vi "BRig_dataExp_T_Reward_min_L.vi"() -> (2 "output_Tcycle_Reward_min_L":i32)   [LabVIEW 2014]
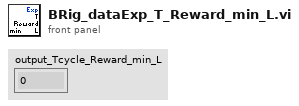
[diagram p1: front panel]
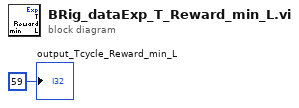
[diagram p0: block diagram]
diagram:
  "output_Tcycle_Reward_min_L" <- 59 ("output_iBlock")
